vi "Send command.vi"(4 "error in":errorcluster, 5 "Command":T1, 6 "F-70 parameters in":T2 {"Last updated" format="%<%d/%m/%Y %H:%M:%S>T"; "State of operation" items=["Local Off", "Local On", "Remote Off", "Remote On", "Cold head Run", "Cold head pause", "Fault Off", "Oil Fault Off"]; "Return pressure (PSIG)" scale=0.0..200.0; "Water in Tmp (°C)" scale=0.0..100.0; "Water out Tmp (°C)" scale=0.0..100.0; "He discharge Tmp (°C)" scale=0.0..100.0}, 7 "VISA resource in":refnum<visa-resource-name>) -> (0 "error out":errorcluster, 2 "F-70 parameters in 2":T2 {"Last updated" format="%<%d/%m/%Y %H:%M:%S>T"; "State of operation" items=["Local Off", "Local On", "Remote Off", "Remote On", "Cold head Run", "Cold head pause", "Fault Off", "Oil Fault Off"]; "Return pressure (PSIG)" scale=0.0..200.0; "Water in Tmp (°C)" scale=0.0..100.0; "Water out Tmp (°C)" scale=0.0..100.0; "He discharge Tmp (°C)" scale=0.0..100.0}, 3 "VISA resource out":refnum<visa-resource-name>)   [LabVIEW 2021, in "F-70 driver.lvlib"]
doc: "Sends a command and processes a response from the compressor into F-70 parameters cluster.\n\nTEA- read TEmperature All [°C]; PRA- read PRessure All [PSIG]; STA- read STAtus bits; ID1- read FW and elapsed hours; ON1- run compressor and cold head; RS1- ReSet fault indications; OFF- stop compressor and cold head; CHP- Cold Head Pause; CHR- Cold Head Runa; POF cold head Pause OFF; TE1- Compressor capsule helium discharge temperature; TE2 - Water outlet temperature; TE3 - Water inlet temperature; TE4- Inactive (\"000\"); PR1- compressor return pressure; PR2- Inactive (\"000\")"
uses:
  F-70 driver.lvlib
  F-70 parameters.ctl
  Commands.ctl
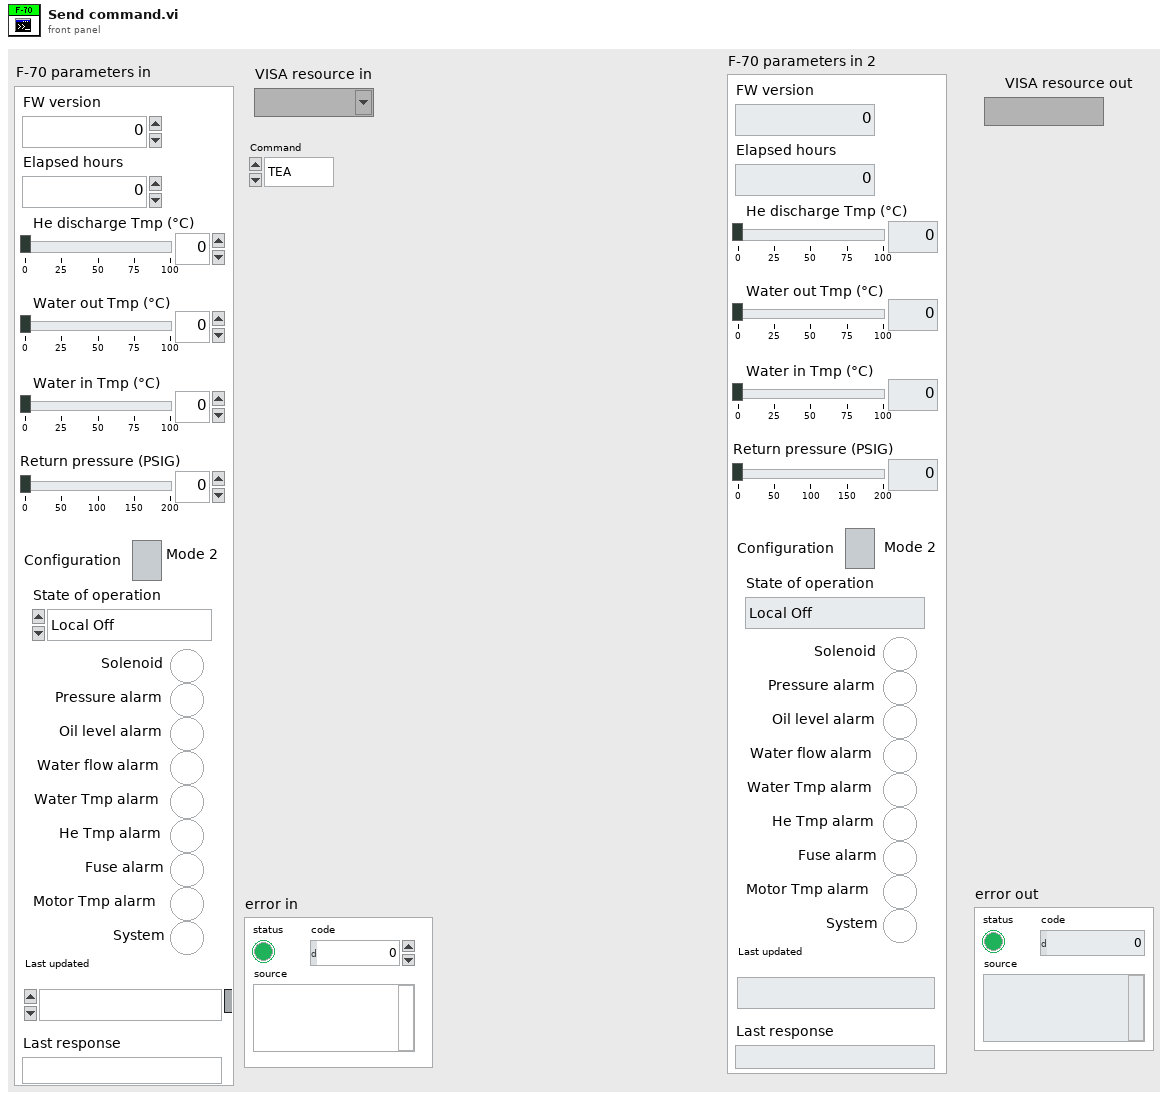
[diagram p1: front panel]
types:
  T1 = typedef "F-70 driver.lvlib/Commands.ctl" = enum16{"TEA", "PRA", "STA", "ID1", "ON1", "RS1", "CHP", "OFF", "CHR", "POF", "TE1", "TE2", "TE3", "TE4", "PR1", "PR2", "???"}
  T2 = typedef "F-70 driver.lvlib/F-70 parameters.ctl" = cluster{"FW version":dbl, "Elapsed hours":dbl, "He discharge Tmp (°C)":dbl, "Water out Tmp (°C)":dbl, "Water in Tmp (°C)":dbl, "Return pressure (PSIG)":dbl, "Configuration":bool, "State of operation":u16, "Solenoid":bool, "Pressure alarm":bool, "Oil level alarm":bool, "Water flow alarm":bool, "Water Tmp alarm":bool, "He Tmp alarm":bool, "Fuse alarm":bool, "Motor Tmp alarm":bool, "System":bool, "Last updated":timestamp, "Last response":string}
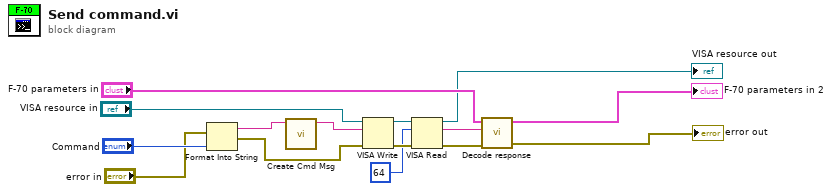
[diagram p0: block diagram]
diagram:
  n1 = Format Into String(error in="error in", "Command") -> (resulting string=w8:string, error out=w7:errorcluster)  [unwired: 2 in]
  n2 = call "Create Cmd Msg.vi"("command"=w8) -> ("complete message"=w4:string)  [unwired: 10 in]
  n3 = VISA Write(VISA resource name="VISA resource in", write buffer=w4, error in (no error)=w7) -> (VISA resource name out=w3:refnum<visa-resource-name>, error out=w6:errorcluster)  [unwired: 1 out]
  n4 = VISA Read(VISA resource name=w3, byte count=u32 64, error in (no error)=w6) -> (VISA resource name out=→"VISA resource out":refnum<visa-resource-name>, read buffer=w1:string, error out=w5:errorcluster)  [unwired: 1 out]
  n5 = call "Decode response.vi"("error in"=w5, "response in"=w1, "F-70 parameters in"="F-70 parameters in") -> ("error out"=→"error out":errorcluster, "F-70 parameters out"=→"F-70 parameters in 2":T2)  [unwired: 7 in]
